vi "Check-Active-filters.vi"(8 "error in":errorcluster, 9 "Available filters":T1[](array[typedef])=[enum."Average intensity [0-255]", enum."Peak intensity [0-255]", enum."Melt-pool size [mm²]", enum."Melt-pool aspect ratio []", enum."Melt-pool fragments []", enum."Melt-pool position X [pixel]", enum."Melt-pool position Y [pixel]", enum."Average temperature [°C]", enum."Max. temperature [°C]", enum."Min. temperature [°C]", enum."Std. dev. temperature [°C]"], 11 "Filter params. ref. in":refnum<data-value>) -> (0 "error IO":errorcluster, 3 "Filter params. ref.":refnum<data-value>, 5 "Passed?":bool)   [LabVIEW 2013, in "CameraVision.lvlib" / "CV-Filter.lvclass"]
uses:
  CV-Filter.lvclass
  Filter-characteristic.ctl
  CV-Filter.lvclass/CV-Filter.ctl
  Read Filter array.vi
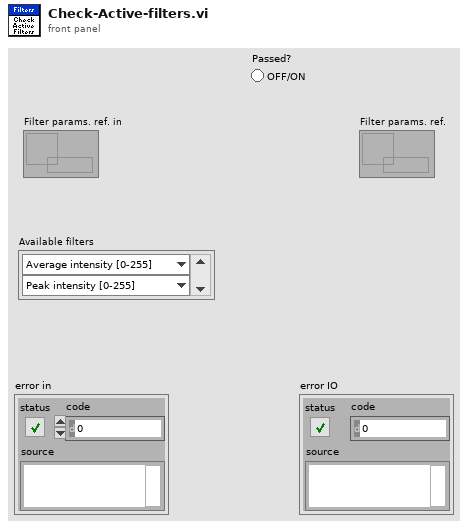
[diagram p1: front panel]
types:
  T1 = typedef "CameraVision.lvlib/CV-Filter.lvclass/Filter-characteristic.ctl" = enum16{"Average intensity [0-255]", "Peak intensity [0-255]", "Melt-pool size [mm²]", "Melt-pool aspect ratio []", "Melt-pool fragments []", "Melt-pool position X [pixel]", "Melt-pool position Y [pixel]", "Average temperature [°C]", "Max. temperature [°C]", "Min. temperature [°C]", "Std. dev. temperature [°C]"}
  T2 = typedef "CameraVision.lvlib/Filter.lvclass/Filter-settings.ctl" = cluster{"Characteristic":T3, "Monitor":bool, "Min.":dbl, "Max.":dbl, "Min. Thres.":dbl, "Min. Dur.":u16, "Report":bool}
  T3 = typedef "CameraVision.lvlib/Filter.lvclass/Filter-characteristic.ctl" = enum16{"Average intensity [0-255]", "Peak intensity [0-255]", "Melt-pool size [mm²]", "Melt-pool aspect ratio []", "Melt-pool fragments []", "Melt-pool position X [pixel]", "Melt-pool position Y [pixel]", "Average temperature [°C]", "Max. temperature [°C]", "Min. temperature [°C]", "Std. dev. temperature [°C]"}
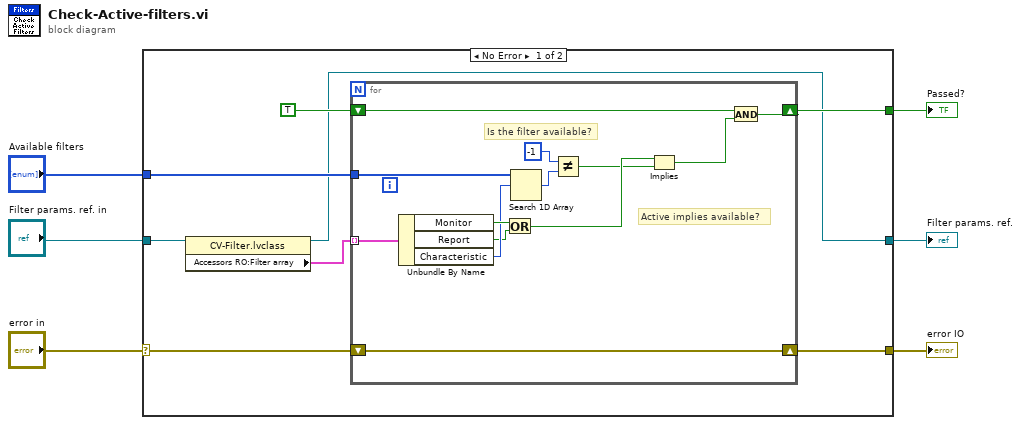
[diagram p0: block diagram]
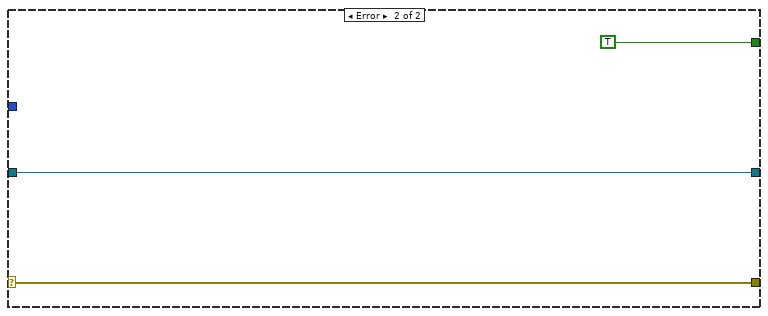
[diagram p2: hidden frame]
diagram:
  n1 = case shown="No Error" "error in" {
    selector: "error in" -> [w13 w30]
    tunnel: [w14 w30] -> w6
    tunnel: "Filter params. ref. in" -> [w9 w28]
    tunnel: "Available filters" -> [w12 _]
    tunnel: [w10 TRUE] -> w3
    tunnel: [w7 w28] -> w1
    frame No Error {
      n2 = property class="CV-Filter.lvclass"(reference=w9) -> (reference out=w7:refnum<data-value>, "Accessors RO:Filter array"=w8:T2[])  [unwired: 1 in, 1 out]
      n3 = for {
        tunnel: w8 -> [w27] mode=indexing
        shift-right: [w15] -> w14
        shift-left: w13 -> [w15]
        tunnel: w12 -> [w25]
        shift-right: [w17] -> w10
        shift-left: TRUE -> [w18]
        # "Active implies available?"
        # "Is the filter available?"
        n4 = Unbundle By Name(w27) -> ("Monitor"=w26:bool, "Report"=w21:bool, "Characteristic"=w24:T3)
        n5 = Or(x=w26, y=w21) -> (x .or. y?=w20:bool)
        n6 = Search 1D Array(1D array=w25, element=w24) -> (index of element=w23:i32)  [unwired: 1 in]
        n7 = Not Equal?(x=-1, y=w23) -> (x != y?=w19:bool)
        n8 = Implies(1:w19, 2:w20) -> (0:w16:bool)
        n9 = And(x=w18, y=w16) -> (x .and. y?=w17:bool)
      }
    }
    frame Error {
    }
  }
  "error IO" <- w6
  "Passed?" <- w3
  "Filter params. ref." <- w1
